vi "AOTF_ETL3_mirror_waveplate_control.vi"() -> ()   [LabVIEW 2017]
uses:
  <vilib>/DAQmx/write.llb/DAQmx Write (Analog DBL 1Chan 1Samp).vi
  <vilib>/DAQmx/write.llb/DAQmx Write (Analog 1D DBL NChan 1Samp).vi
  <vilib>/DAQmx/create/channels.llb/DAQmx Create Channel (AO-Voltage-Basic).vi
  <vilib>/DAQmx/miscellaneous.llb/DAQmx Fill In Error Info.vi
  <vilib>/Utility/file.llb/Read Delimited Spreadsheet (DBL).vi
panel:
  in  "Waveplate Voltage Profiles\n<Read from \"waveplate.csv\">":T1(radio)
  out "Diopter":dbl
  out "Focal Distance (um)":dbl
  in  "ETL3 (v)  (4.76V allows light passing through unaltered.)":dbl(slide)=4.76 caption="ETL3 (dpt)" min=-12.029999732971191 max=16.450000762939453 step=0.009999999776482582 scale=0.0..10.0
  in  "Y Multiplier":dbl=1.0 format="%#_13g"
  in  "X Multiplier":dbl=-1.0 format="%#_13g"
  in  "Mirror 1 Combined Movement (V) (X * X Multiplier + Y * Y Multiplier)":dbl(slide) min=-10.0 max=10.0 step=0.01 scale=-10.0..10.0
  in  "Mirror 1 - Y (v)":dbl(slide) min=-10.0 max=10.0 step=0.01 scale=-10.0..10.0
  in  "Mirror 1 - X (v)":dbl(slide) min=-10.0 max=10.0 step=0.01 scale=-10.0..10.0
  in  "561 (0-10v)":dbl min=0.0 max=10.0 format="%#_13g"
  in  "488 (0-10v)":dbl min=0.0 max=10.0 format="%#_13g"
  in  "Blanking(0-10v)\n(10 for full power)":dbl=10.0 min=0.0 max=10.0 step=0.1 format="%#_13g"
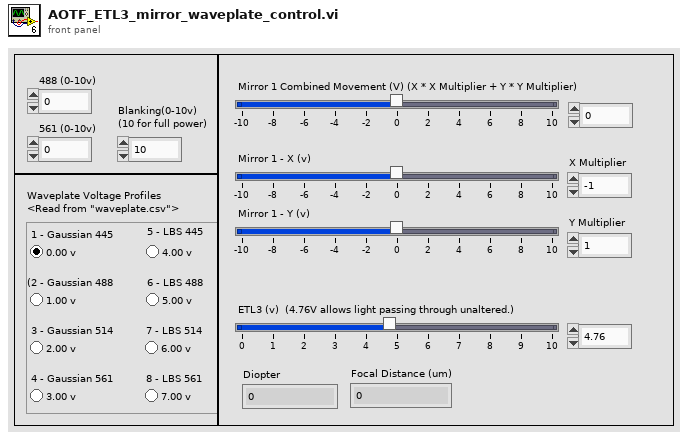
[diagram p1: front panel]
types:
  T1 = enum32{"1 - Gaussian 445", "(2 - Gaussian 488", "3 - Gaussian 514", "4 - Gaussian 561", "5 - LBS 445", "6 - LBS 488", "7 - LBS 514", "8 - LBS 561"}
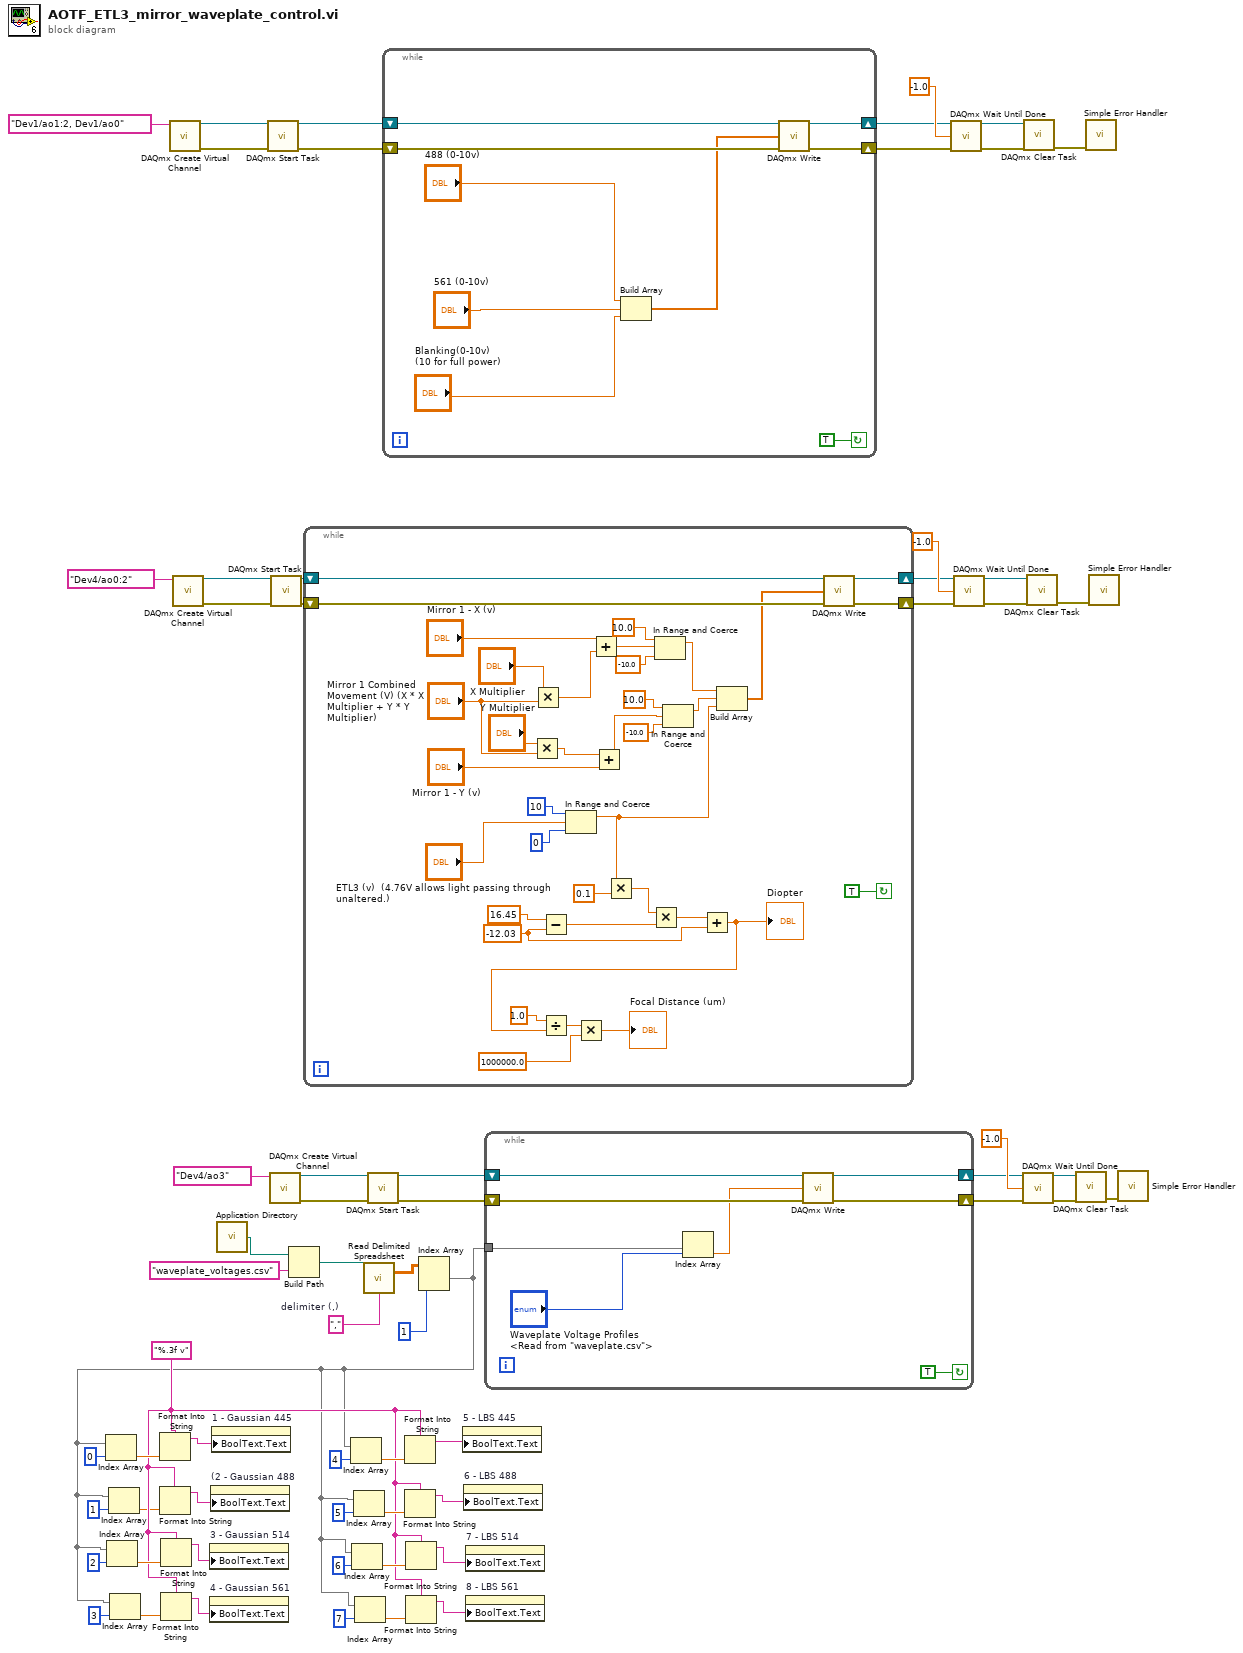
[diagram p0: block diagram]
diagram:
  w7 = "%.3f v" ("format string")
  w32 = ","  # delimiter (,)
  n1 = call-poly <vilib>:"DAQmx Create Virtual Channel.vi"("physical channels"=tag "Dev1/ao1:2, Dev1/ao0") -> ("task out"=w58:refnum<k21>, "error out"=w57:errorcluster)  [unwired: 13 in]
  n2 = call-poly <vilib>:"DAQmx Create Virtual Channel.vi"("physical channels"=tag "Dev4/ao0:2") -> ("task out"=w47:refnum<k21>, "error out"=w46:errorcluster)  [unwired: 13 in]
  n3 = call <vilib>:"Application Directory.vi"() -> ("Application Directory"=w31:path)
  n4 = call <vilib>:"DAQmx Start Task.vi"("task/channels in"=w58, "error in"=w57) -> ("task out"=w60:refnum<k21>, "error out"=w59:errorcluster)  [unwired: 12 in]
  n5 = call-poly <vilib>:"DAQmx Create Virtual Channel.vi"("physical channels"=tag "Dev4/ao3") -> ("task out"=w36:refnum<k21>, "error out"=w35:errorcluster)  [unwired: 13 in]
  n6 = call <vilib>:"DAQmx Start Task.vi"("task/channels in"=w47, "error in"=w46) -> ("task out"=w49:refnum<k21>, "error out"=w48:errorcluster)  [unwired: 12 in]
  n7 = Build Path(base path=w31, name or relative path="waveplate_voltages.csv") -> (appended path=w29:path)
  n8 = while {
    shift-right: [w99] -> w44
    shift-left: w49 -> [w101]
    shift-right: [w98] -> w45
    shift-left: w48 -> [w100]
    stop <- TRUE continue-if-true
    w68 = -12.03 ("x")
    n9 = Multiply(x="Y Multiplier", y="Mirror 1 Combined Movement (V) (X * X Multiplier + Y * Y Multiplier)") -> (x*y=w81:dbl)
    n10 = Multiply(x="X Multiplier", y="Mirror 1 Combined Movement (V) (X * X Multiplier + Y * Y Multiplier)") -> (x*y=w94:dbl)
    n11 = Subtract(x=16.45 ("y"), y=w68) -> (x-y=w70:dbl)
    n12 = In Range and Coerce(upper limit=10, x="ETL3 (v)  (4.76V allows light passing through unaltered.)", lower limit=0) -> (coerced(x)=w66:dbl)  [unwired: 1 out]
    n13 = Add(x="Mirror 1 - X (v)", y=w94) -> (x+y=w91:dbl)
    n14 = Add(x=w81, y="Mirror 1 - Y (v)") -> (x+y=w85:dbl)
    n15 = Multiply(x=w66, y=0.1) -> (x*y=w71:dbl)
    n16 = Multiply(x=w71, y=w70) -> (x*y=w69:dbl)
    n17 = In Range and Coerce(upper limit=10.0, x=w91, lower limit=-10.0) -> (coerced(x)=w88:dbl)  [unwired: 1 out]
    n18 = In Range and Coerce(upper limit=10.0, x=w85, lower limit=-10.0) -> (coerced(x)=w84:dbl)  [unwired: 1 out]
    n19 = Add(x=w69, y=w68) -> (x+y=w67:dbl)
    "Diopter" <- w67
    n20 = Divide(x=1.0, y=w67) -> (x/y=w79:dbl)
    n21 = Multiply(x=w79, y=1000000.0) -> (x*y=→"Focal Distance (um)":dbl)
    n22 = Build Array(w88, w84, w66) -> (w97:dbl[])
    n23 = call-poly <vilib>:"DAQmx Write.vi"("task/channels in"=w101, "data"=w97, "error in"=w100) -> ("task out"=w99:refnum<k21>, "error out"=w98:errorcluster)  [unwired: 10 in, 1 out]
  }
  n24 = call-poly <vilib>:"Read Delimited Spreadsheet.vi"("file path (dialog if empty)"=w29, "delimiter (\\t)"=w32) -> ("all rows"=w4:dbl[][])  [unwired: 8 in, 5 out]
  n25 = call <vilib>:"DAQmx Start Task.vi"("task/channels in"=w36, "error in"=w35) -> ("task out"=w38:refnum<k21>, "error out"=w37:errorcluster)  [unwired: 12 in]
  n26 = while {
    shift-right: [w108] -> w55
    shift-left: w60 -> [w110]
    shift-right: [w107] -> w56
    shift-left: w59 -> [w109]
    stop <- TRUE continue-if-true
    n27 = Build Array("488 (0-10v)", "561 (0-10v)", "Blanking(0-10v)\n(10 for full power)") -> (w106:dbl[])
    n28 = call-poly <vilib>:"DAQmx Write.vi"("task/channels in"=w110, "data"=w106, "error in"=w109) -> ("task out"=w108:refnum<k21>, "error out"=w107:errorcluster)  [unwired: 10 in, 1 out]
  }
  n29 = Index Array(array=w4, index (row)=1) -> (element=w1:dbl[])  [unwired: 1 in]
  n30 = Index Array(array=w1, index=0) -> (element=w16:dbl)
  n31 = Index Array(array=w1, index=2) -> (element=w18:dbl)
  n32 = Index Array(array=w1, index=1) -> (element=w2:dbl)
  n33 = Index Array(array=w1, index=3) -> (element=w17:dbl)
  n34 = Format Into String(format string=w7, w16) -> (resulting string=w15:string)  [unwired: 2 in, 1 out]
  n35 = Format Into String(format string=w7, w2) -> (resulting string=w14:string)  [unwired: 2 in, 1 out]
  n36 = Format Into String(format string=w7, w18) -> (resulting string=w13:string)  [unwired: 2 in, 1 out]
  n37 = Format Into String(format string=w7, w17) -> (resulting string=w12:string)  [unwired: 2 in, 1 out]
  n38 = property on="3 - Gaussian 514" class="Bool (strict)"("BoolText.Text"=w13) -> ()  [unwired: 2 in, 2 out]
  n39 = property on="4 - Gaussian 561" class="Bool (strict)"("BoolText.Text"=w12) -> ()  [unwired: 2 in, 2 out]
  n40 = property on="(2 - Gaussian 488" class="Bool (strict)"("BoolText.Text"=w14) -> ()  [unwired: 2 in, 2 out]
  n41 = property on="1 - Gaussian 445" class="Bool (strict)"("BoolText.Text"=w15) -> ()  [unwired: 2 in, 2 out]
  n42 = Index Array(array=w1, index=4) -> (element=w22:dbl)
  n43 = Index Array(array=w1, index=6) -> (element=w26:dbl)
  n44 = Index Array(array=w1, index=5) -> (element=w21:dbl)
  n45 = Index Array(array=w1, index=7) -> (element=w25:dbl)
  n46 = Format Into String(format string=w7, w22) -> (resulting string=w6:string)  [unwired: 2 in, 1 out]
  n47 = Format Into String(format string=w7, w21) -> (resulting string=w5:string)  [unwired: 2 in, 1 out]
  n48 = Format Into String(format string=w7, w26) -> (resulting string=w24:string)  [unwired: 2 in, 1 out]
  n49 = Format Into String(format string=w7, w25) -> (resulting string=w23:string)  [unwired: 2 in, 1 out]
  n50 = property on="5 - LBS 445" class="Bool (strict)"("BoolText.Text"=w6) -> ()  [unwired: 2 in, 2 out]
  n51 = property on="6 - LBS 488" class="Bool (strict)"("BoolText.Text"=w5) -> ()  [unwired: 2 in, 2 out]
  n52 = property on="7 - LBS 514" class="Bool (strict)"("BoolText.Text"=w24) -> ()  [unwired: 2 in, 2 out]
  n53 = property on="8 - LBS 561" class="Bool (strict)"("BoolText.Text"=w23) -> ()  [unwired: 2 in, 2 out]
  n54 = while {
    shift-right: [w116] -> w33
    shift-left: w38 -> [w118]
    shift-right: [w115] -> w34
    shift-left: w37 -> [w117]
    tunnel: w1 -> [w112]
    stop <- TRUE continue-if-true
    n55 = Index Array(array=w112, index="Waveplate Voltage Profiles\n<Read from \"waveplate.csv\">") -> (element=w111:dbl)
    n56 = call-poly <vilib>:"DAQmx Write.vi"("task/channels in"=w118, "data"=w111, "error in"=w117) -> ("task out"=w116:refnum<k21>, "error out"=w115:errorcluster)  [unwired: 10 in, 1 out]
  }
  n57 = call <vilib>:"DAQmx Wait Until Done.vi"("task/channels in"=w55, "timeout (sec)"=-1.0, "error in"=w56) -> ("task out"=w64:refnum<k21>, "error out"=w63:errorcluster)  [unwired: 11 in]
  n58 = call <vilib>:"DAQmx Wait Until Done.vi"("task/channels in"=w44, "timeout (sec)"=-1.0, "error in"=w45) -> ("task out"=w53:refnum<k21>, "error out"=w52:errorcluster)  [unwired: 11 in]
  n59 = call <vilib>:"DAQmx Wait Until Done.vi"("task/channels in"=w33, "timeout (sec)"=-1.0, "error in"=w34) -> ("task out"=w42:refnum<k21>, "error out"=w41:errorcluster)  [unwired: 11 in]
  n60 = call <vilib>:"DAQmx Clear Task.vi"("task in"=w64, "error in"=w63) -> ("error out"=w65:errorcluster)  [unwired: 13 in]
  n61 = call <vilib>:"DAQmx Clear Task.vi"("task in"=w53, "error in"=w52) -> ("error out"=w54:errorcluster)  [unwired: 13 in]
  n62 = call <vilib>:"DAQmx Clear Task.vi"("task in"=w42, "error in"=w41) -> ("error out"=w43:errorcluster)  [unwired: 13 in]
  n63 = call <vilib>:"Simple Error Handler.vi"("error in (no error)"=w65) -> ()  [unwired: 4 in, 5 out]
  n64 = call <vilib>:"Simple Error Handler.vi"("error in (no error)"=w54) -> ()  [unwired: 4 in, 5 out]
  n65 = call <vilib>:"Simple Error Handler.vi"("error in (no error)"=w43) -> ()  [unwired: 4 in, 5 out]
